vi "Varian_PUMP_STOP.vi"(5 "APX:AP1Trubo_STOP":bool, 7 "PV Name":string, 8 "error in (no error)":errorcluster, 9 "APX:AP1STurboS":dbl, 11 "VISA Refnum in":refnum<visa-resource-name>) -> (0 "error out":errorcluster, 3 "VISA Refnum out":refnum<visa-resource-name>)   [LabVIEW 2015]
uses:
  <userlib>/caLab/Private/Put_DBL_PV.vi
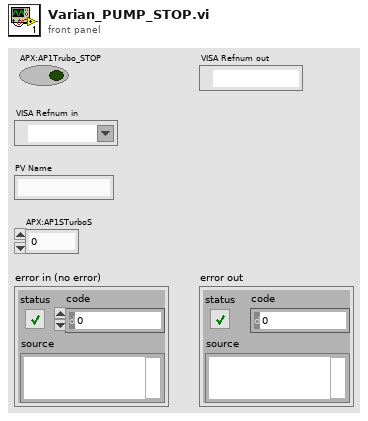
[diagram p1: front panel]
types:
  T1 = enum16{"START", "STOP", "REMOTE/SERIAL", "REMOTE", "SERIAL", "START/STOP", "PUMP STATUS", "Driving Frequency", "PUMP POWER", "PRESSURE"}
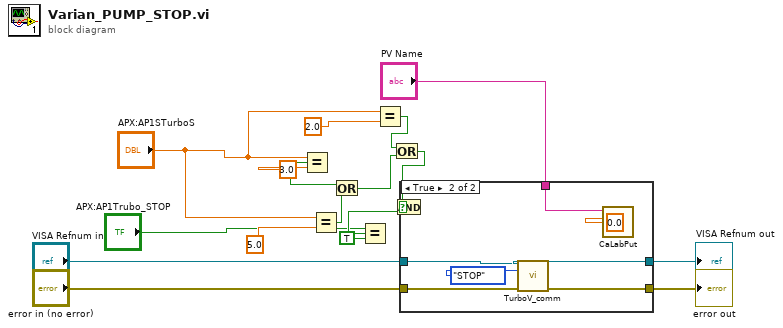
[diagram p0: block diagram]
diagram:
  n1 = Equal?(x="APX:AP1STurboS", y=3.0) -> (x = y?=w10:bool)
  n2 = Equal?(x="APX:AP1STurboS", y=5.0) -> (x = y?=w9:bool)
  n3 = Or(x=w10, y=w9) -> (x .or. y?=w2:bool)
  n4 = Equal?(x="APX:AP1Trubo_STOP", y=TRUE) -> (x = y?=w8:bool)
  n5 = Equal?(x="APX:AP1STurboS", y=2.0) -> (x = y?=w3:bool)
  n6 = Or(x=w3, y=w2) -> (x .or. y?=w1:bool)
  n7 = And(x=w1, y=w8) -> (x .and. y?=w13:bool)
  n8 = case shown="True" w13 {
    tunnel: [w20 w27] -> w16
    tunnel: [w19 w26] -> w17
    tunnel: "VISA Refnum in" -> [w20 w24]
    tunnel: "error in (no error)" -> [w19 w23]
    tunnel: "PV Name" -> [_ w21]
    frame False {
    }
    frame True {
      n9 = call "TurboV_comm.vi"("VISA resource name"=w24, "Command"=T1."STOP", "error in (no error)"=w23) -> ("VISA resource name out"=w27:refnum<visa-resource-name>, "error out"=w26:errorcluster)  [unwired: 10 in, 1 out]
      n10 = call-poly <userlib>:"CaLabPut.vi"("Value"=0.0, "PV Name"=w21) -> ()  [unwired: 6 in, 4 out]
    }
  }
  "error out" <- w17
  "VISA Refnum out" <- w16
